vi "IR Scan.vi"() -> ()   [LabVIEW 2013]
uses:
  <vilib>/FPGAPlugInAG/sbRIO-9642/niLvFpga_Open_sbRIO-9642.vi
  <vilib>/rvi/interface/common/dynamic/niFpgaDynamicAddResources.vi
  <vilib>/rvi/interface/common/niFpgaWaitOnOcc.vi
  <vilib>/Utility/error.llb/Error Cluster From Error Code.vi
  <vilib>/rvi/errors/niLvFpgaAdjustHostInterfaceError.vi
  <vilib>/rvi/interface/nirviOpenFPGA/nirviOpenFPGA.xnode
  FPGA Bitfiles/NatesProject1_FPGATarget_FPGAConfig_gDHlPw7zMRU.lvbitx
  FPGA Config.vi
  <vilib>/rvi/interface/nirviReadWriteControl/nirviReadWriteControl.xnode
  NiFpgaLv.dll
  <vilib>/rvi/interface/Simulation/niFpgaSimulationCallBeginRW.vi
  <vilib>/robotics/Utilities/Scan Angles/NI_Robotics_Scan Angles.lvlib
panel:
  out "Sensor Data":cluster{"angles (deg)":dbl[], "distances":dbl[]}(graph)
  out "Waveform Chart":dbl(graph)
  out "Front Sensor\nDistance\n(cm)":dbl(slide) scale=0.0..150.0
  in  "stop":bool
  out "ModA/AI0":fxp<+/-,26,5>
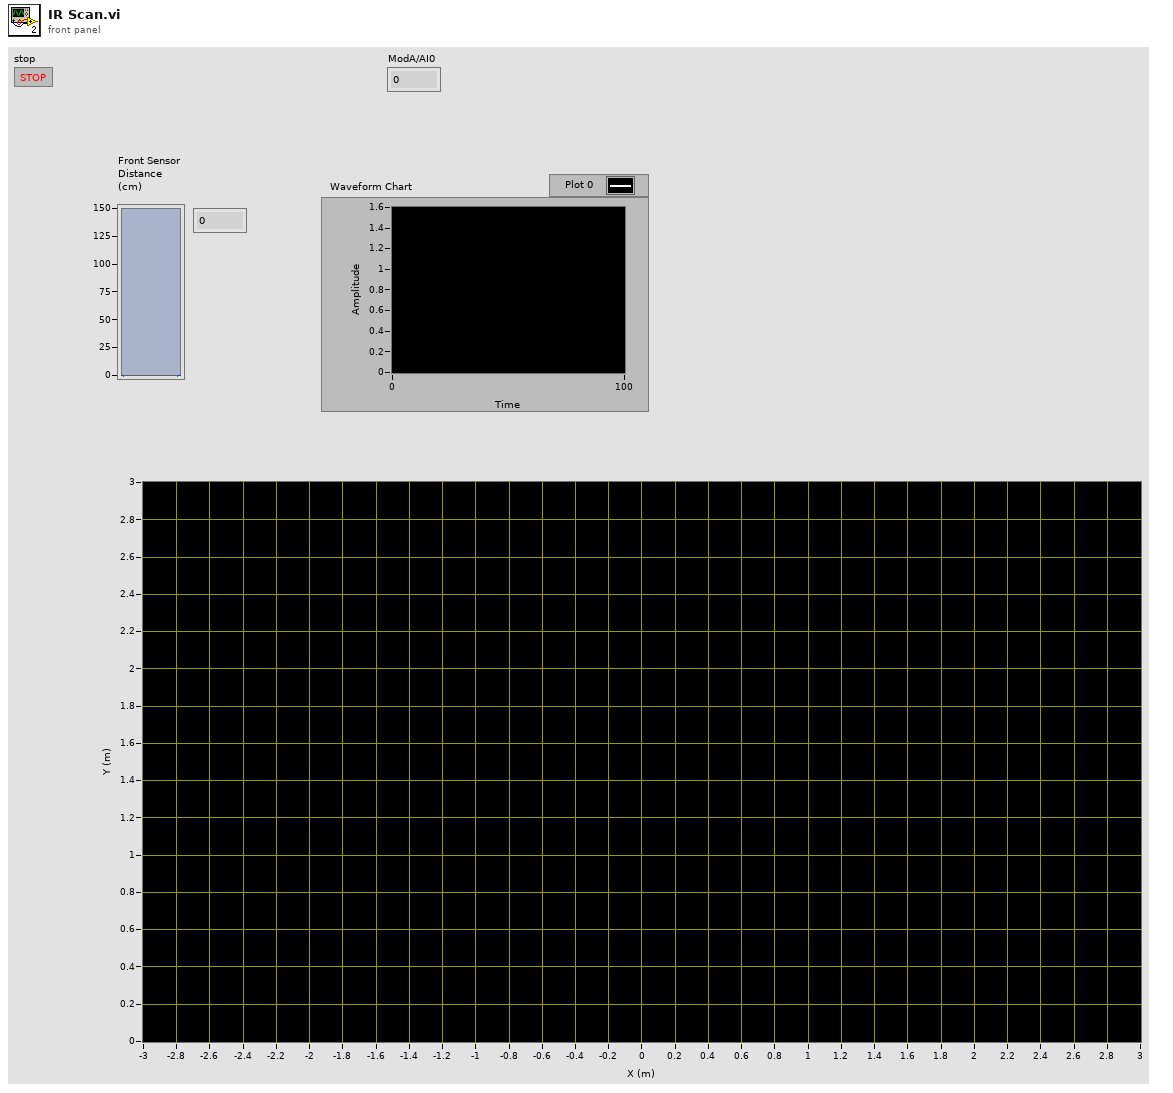
[diagram p1: front panel]
types:
  T1 = typedef "NI_Robotics_Scan Angles.lvlib/Scan Angle Data.ctl" = cluster{"angles":dbl[], "distances":dbl[], "current index":i32, "previous index":i32}
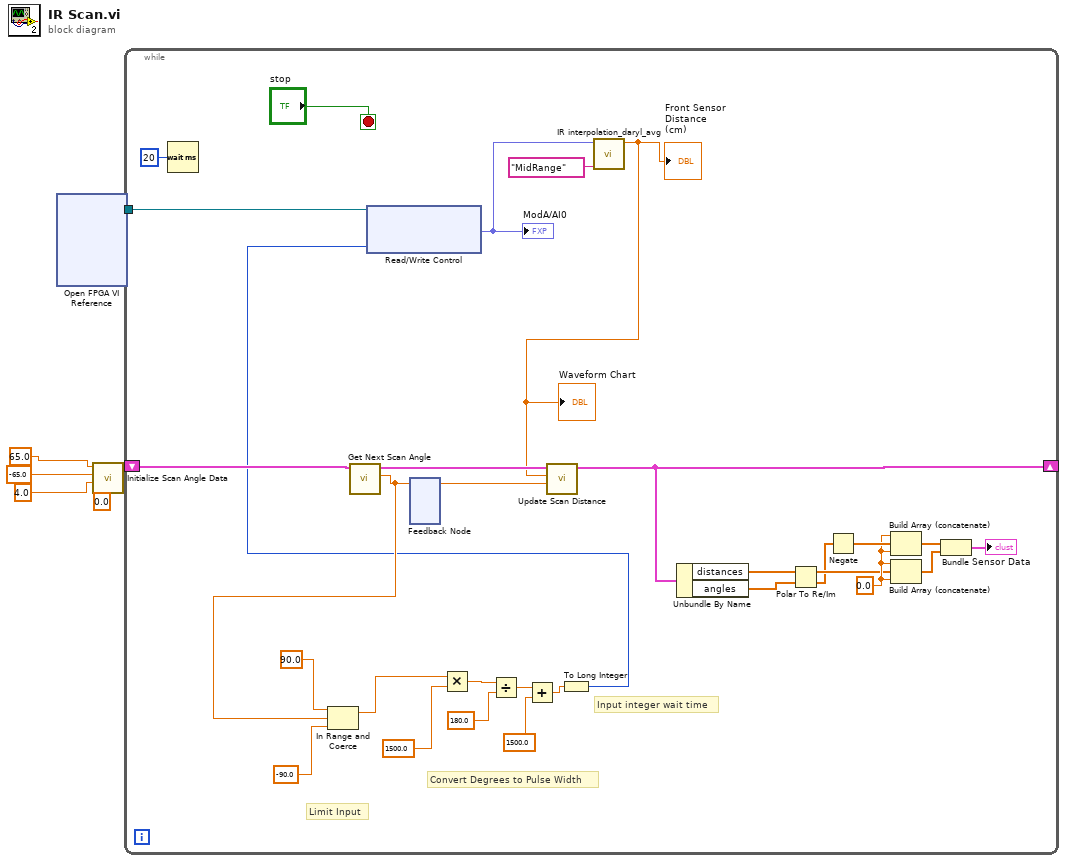
[diagram p0: block diagram]
diagram:
  n1 = xnode "Open FPGA VI Reference"() -> ("FPGA VI Reference Out"=w6:refnum<k20>)  [unwired: 2 in, 1 out]
  n2 = call <vilib>:"Initialize Scan Angle Data.vi"("initial angle (0)"=0.0, "scan angle"=4.0, "min angle"=-65.0, "max angle"=65.0) -> ("scan angles"=w1:T1)  [unwired: 6 in, 1 out]
  n3 = while {
    tunnel: w6 -> [w33]
    shift-right: [w8] -> _
    shift-left: w1 -> [w30]
    stop <- "stop" stop-if-true
    w15 = 0.0 ("element")
    # "Input integer wait time"
    # "Convert Degrees to Pulse Width"
    # "Limit Input"
    n4 = Wait (ms)(milliseconds to wait=u32 20) -> ()  [unwired: 1 out]
    n5 = call <vilib>:"Get Next Scan Angle.vi"("scan angles in"=w30) -> ("new angle"=w19:dbl, "scan angles out"=w32:T1)  [unwired: 9 in]
    n6 = In Range and Coerce(upper limit=90.0, x=w19, lower limit=-90.0) -> (coerced(x)=w28:dbl)  [unwired: 1 out]
    n7 = feedback #1() -> (w31:dbl)  [unwired: 1 in]
    n8 = feedback-in #1(w19) -> ()
    n9 = Multiply(x=w28, y=1500.0) -> (x*y=w25:dbl)
    n10 = Divide(x=w25, y=180.0) -> (x/y=w22:dbl)
    n11 = Add(x=w22, y=1500.0) -> (x+y=w21:dbl)
    n12 = To Long Integer(number=w21) -> (32bit integer=w18:i32)
    n13 = xnode "Read/Write Control"("FPGA VI Reference In"=w33, "Pulse Width(uSec)"=w18) -> ("ModA/AI1"=w35:fxp<+/-,26,5>)  [unwired: 1 in, 2 out]
    "ModA/AI0" <- w35
    n14 = call "IR interpolation_daryl_avg.vi"("IR Sensor Type"="MidRange", "x value"=w35) -> ("interpolation value"=w29:dbl)  [unwired: 9 in]
    "Front Sensor\nDistance\n(cm)" <- w29
    "Waveform Chart" <- w29
    n15 = call <vilib>:"Update Scan Distance.vi"("scan angle"=w31, "new scan distance"=w29, "scan angles in"=w32) -> ("scan angles out"=w8:T1)  [unwired: 8 in]
    n16 = Unbundle By Name(w8) -> ("distances"=w10:dbl[], "angles"=w9:dbl[])
    n17 = Polar To Re/Im(2:w9, 3:w10) -> (0:w12:dbl[], 1:w13:dbl[])
    n18 = Negate(x=w12) -> (-x=w17:dbl[])
    n19 = Build Array (concatenate)(w15, w17, w15) -> (w16:dbl[])
    n20 = Build Array (concatenate)(w15, w13, w15) -> (w14:dbl[])
    n21 = Bundle(w16, w14) -> (→"Sensor Data":cluster{dbl[], dbl[]})  [unwired: 1 in]
  }
